vi "analogReadout.vi"() -> ()   [LabVIEW 2017]
uses:
  <vilib>/rvi/Emulation/niFpgaGetClockAttributes.vi
  <vilib>/rvi/Emulation/niFpgaSctlEmulationGetInTimedLoop.vi
  <vilib>/rvi/Emulation/niFpgaEmulationReportErrorSimple.vi
  <vilib>/rvi/eio/common/nirviEmuTemplateMethod_errors.vi
  <vilib>/rvi/interface/RandomDataEmulation/niFpgaRandomDataHandleErrors.vi
  <vilib>/rvi/Emulation/niFpgaCriticalErrorInLSC.vi
  <vilib>/eio/EIONode/EIONode.xnode
  <vilib>/rvi/DataTransferAndStorage/Container/XNode/niFpgaContainer.xnode
  <vilib>/rvi/interface/RandomDataEmulation/nirviRandomDataFpgaReadWriteTemplate.vi
panel:
  out "timeout":bool
  in  "dT":i16
  in  "write to buffer":bool
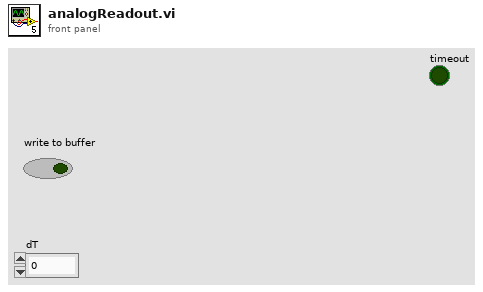
[diagram p1: front panel]
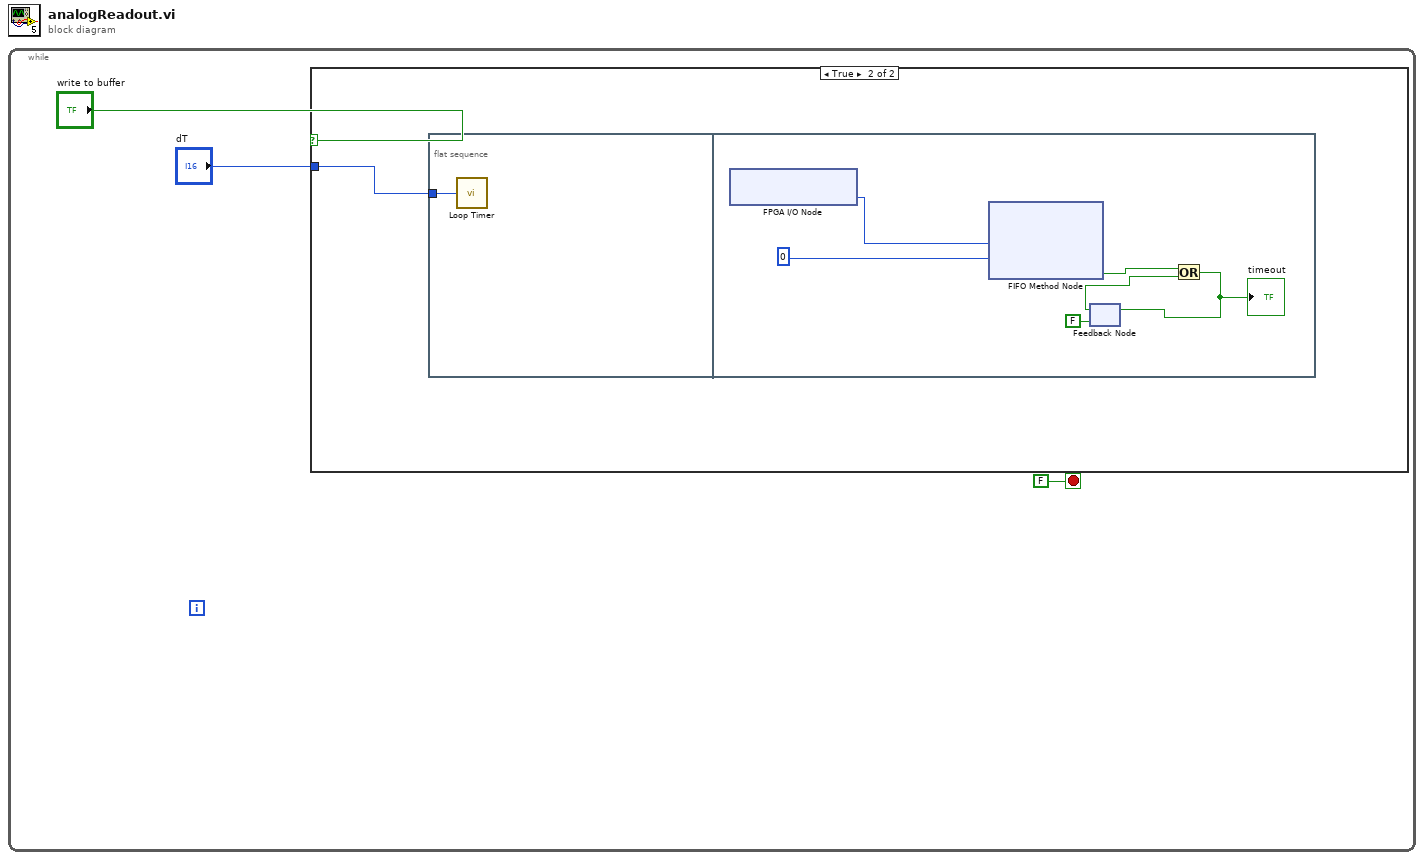
[diagram p0: block diagram]
diagram:
  n1 = while {
    stop <- FALSE stop-if-true
    n2 = case shown="True" "write to buffer" {
      tunnel: "dT" -> [_ w4]
      frame False {
      }
      frame True {
        n3 = flat-sequence {
          tunnel: w4 -> [w5]
          frame #0 {
            n4 = call "Loop Timer"("Count(uSec)"=w5) -> ()  [unwired: 1 out]
          }
          frame #1 {
            n5 = xnode "FPGA I/O Node"() -> ("Connector0/AI4"=w11:i16)  [unwired: 1 in, 1 out]
            n6 = xnode ("FIFO Method Node")("Element"=w11, "Timeout"=0) -> ("Timed Out?"=w9:bool)  [unwired: 1 in, 1 out]
            n7 = feedback #1(FALSE) -> (w7:bool)
            n8 = Or(x=w9, y=w7) -> (x .or. y?=w8:bool)
            "timeout" <- w8
            n9 = feedback-in #1(w8) -> ()
          }
        }
      }
    }
  }
